vi "Delete Thing.vi"(8 "error in (no error)":errorcluster, 9 "Expected Version":i32, 10 "Name":string, 11 "IoT Session in":refnum<class "IoT Session.lvclass">) -> (0 "error out":errorcluster, 3 "IoT Session out":refnum<class "IoT Session.lvclass">)   [LabVIEW 2015, in "NI_AWS_IoT.lvlib" / "IoT Session.lvclass"]
uses:
  IoT Session.lvclass
  Core/HTTP Request/Request Options.ctl
  Core/HTTP Request/Name Value Pair.ctl
  Core/HTTP Request/Region handling.ctl
  Core/HTTP Request/URL formatting.ctl
  Core/HTTP Request/HTTP Request.lvclass
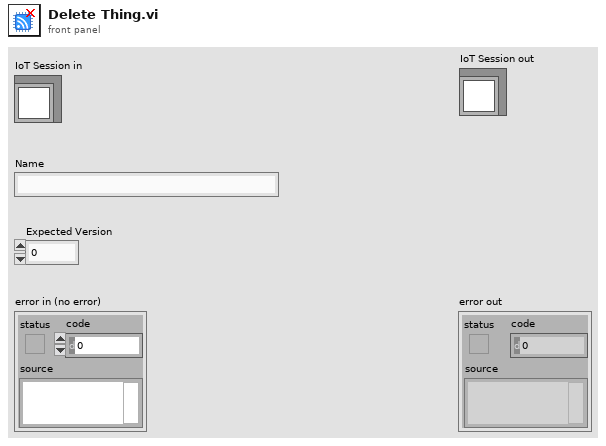
[diagram p1: front panel]
types:
  T1 = typedef "NI_AWS_Core.lvlib/HTTP Request.lvclass/Name Value Pair.ctl" = cluster{"name":string, "value":string}
  T2 = typedef "NI_AWS_Core.lvlib/HTTP Request.lvclass/Request Options.ctl" = cluster{"request headers":T1[], "request parameters":T1[], "request body":string, "region handling":T3, "URL formatting":T4}
  T3 = typedef "NI_AWS_Core.lvlib/HTTP Request.lvclass/Region handling.ctl" = enum16{"use region everywhere", "use region (authentication only)", "use region (URL only)", "ignore region everwhere"}
  T4 = typedef "NI_AWS_Core.lvlib/HTTP Request.lvclass/URL formatting.ctl" = enum16{"region-", "region."}
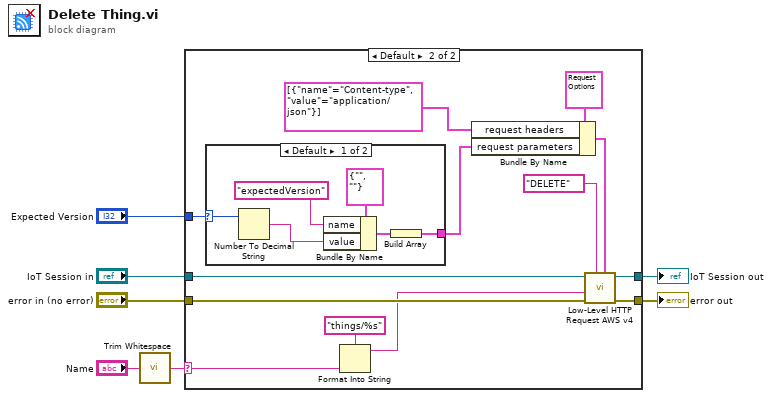
[diagram p0: block diagram]
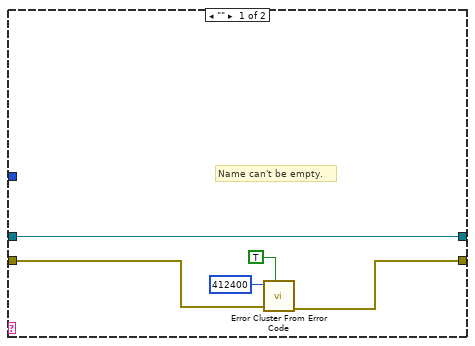
[diagram p2: hidden frame]
diagram:
  n1 = call <vilib>:"Trim Whitespace.vi"("string"="Name") -> ("trimmed string"=w2:string)  [unwired: 1 in]
  n2 = case shown="Default" w2 {
    selector: w2 -> [_ w21]
    tunnel: "error in (no error)" -> [w9 w25]
    tunnel: [w8 w24] -> w6
    tunnel: [w12 w23] -> w5
    tunnel: "IoT Session in" -> [w12 w22]
    tunnel: "Expected Version" -> [_ w14]
    frame "" {
      # "Name can't be empty."
      n3 = call <vilib>:"Error Cluster From Error Code.vi"("show call chain? (False)"=TRUE, "error in (no error)"=w9, "error code (0)"=412400) -> ("error out"=w8:errorcluster)  [unwired: 6 in]
    }
    frame Default {
      n4 = case shown="Default" w14 {
        selector: w14 -> [w27 _]
        tunnel: [w29 _] -> w13
        frame Default {
          n5 = Number To Decimal String(number=w27) -> (decimal integer string=w26:string)  [unwired: 1 in]
          n6 = Bundle By Name(cluster=T1 {"name"="", "value"=""} ("Name Value Pair"), "name"="expectedVersion", "value"=w26) -> (w30:T1)
          n7 = Build Array(w30) -> (w29:T1[])
        }
        frame 0 {
        }
      }
      n8 = Format Into String(format string="things/%s", w21) -> (resulting string=w18:string)  [unwired: 2 in, 1 out]
      n9 = Bundle By Name(cluster=T2 {"request headers"=[], "request parameters"=[], "request body"="", "region handling"=enum."use region everywhere", "URL formatting"=enum."region."} ("Request Options"), "request headers"=T1[] [{"name"="Content-type", "value"="application/json"}], "request parameters"=w13) -> (w16:T2)
      n10 = call "Low-Level HTTP Request AWS v4.vi"("Request Options"=w16, "HTTP-Verb"="DELETE", "error in (no error)"=w25, "URL Suffix"=w18, "AWS Core in"=w22) -> ("error out"=w24:errorcluster, "AWS Core out"=w23:refnum<class "IoT Session.lvclass">)  [unwired: 3 in, 2 out]
    }
  }
  "error out" <- w6
  "IoT Session out" <- w5
